vi "Calculate Uncertainty.vi"(3 "du":dbl, 5 "dL":dbl, 7 "df":dbl, 8 "Linear Density":dbl, 9 "Length":dbl, 10 "Tension":dbl, 11 "Frequency":dbl) -> (0 "dT":dbl)   [LabVIEW 2018]
panel:
  # "Inputs"
  # "Output"
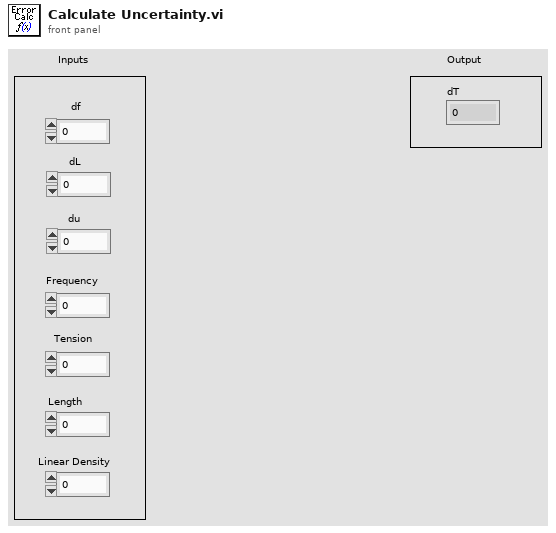
[diagram p1: front panel]
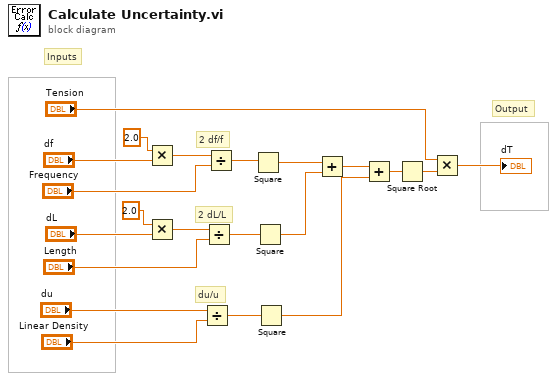
[diagram p0: block diagram]
diagram:
  # "Inputs"
  # "Output"
  # "2 df/f"
  # "2 dL/L"
  # "du/u"
  n1 = Multiply(x=2.0, y="df") -> (x*y=w16:dbl)
  n2 = Multiply(x=2.0, y="dL") -> (x*y=w17:dbl)
  n3 = Divide(x="du", y="Linear Density") -> (x/y=w9:dbl)
  n4 = Divide(x=w17, y="Length") -> (x/y=w10:dbl)
  n5 = Divide(x=w16, y="Frequency") -> (x/y=w11:dbl)
  n6 = Square(x=w11) -> (x^2=w8:dbl)
  n7 = Square(x=w10) -> (x^2=w6:dbl)
  n8 = Square(x=w9) -> (x^2=w5:dbl)
  n9 = Add(x=w8, y=w6) -> (x+y=w7:dbl)
  n10 = Add(x=w7, y=w5) -> (x+y=w4:dbl)
  n11 = Square Root(x=w4) -> (sqrt(x)=w3:dbl)
  n12 = Multiply(x="Tension", y=w3) -> (x*y=→"dT":dbl)
